vi "Configuration Dialog.vi"(8 "error in (no error)":errorcluster, 11 "Error Handler In":refnum<class "Error Handler.lvclass">) -> (0 "error out":errorcluster, 3 "Error Handler Out":refnum<class "Error Handler.lvclass">)   [LabVIEW 2020, in "Error Handler.lvclass"]
uses:
  Error Handler.lvclass
  Error Handler.lvclass/Error Handler.ctl
panel:
  in  "Silent handling?":bool
  in  "Error Log Directory":path
  in  "Cancel":bool
  in  "Commit":bool
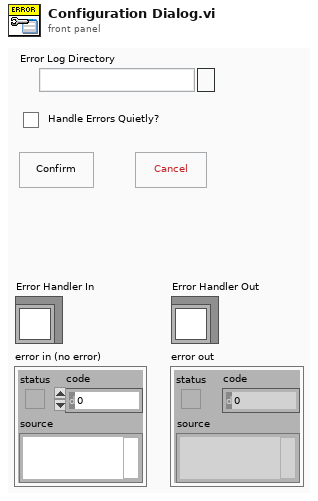
[diagram p1: front panel]
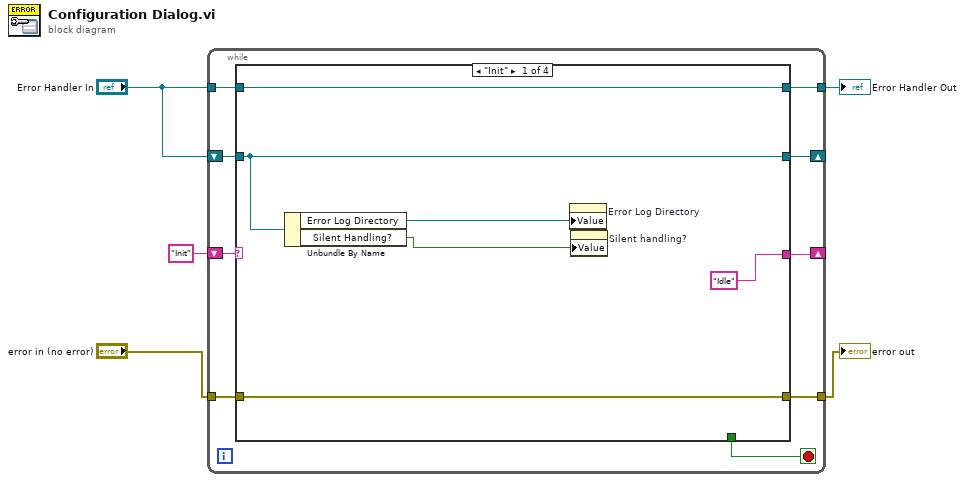
[diagram p0: block diagram]
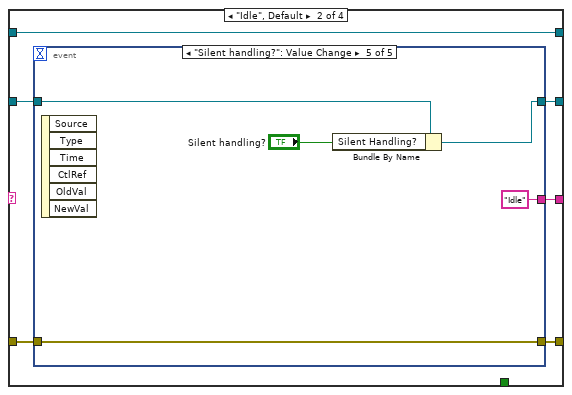
[diagram p2: hidden frame]
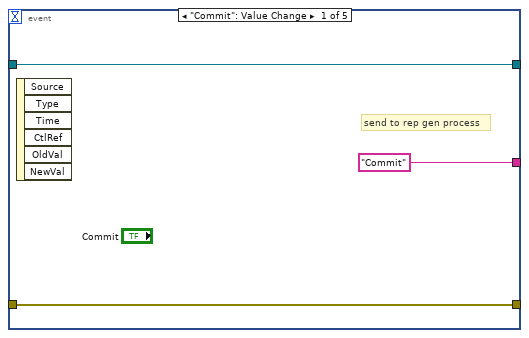
[diagram p3: hidden frame]
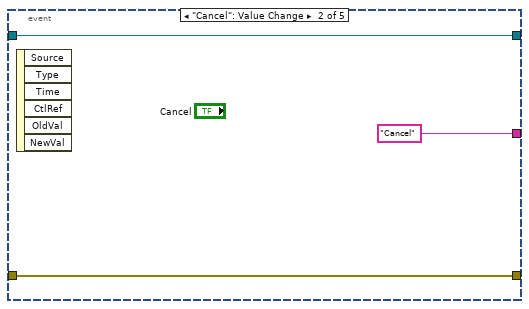
[diagram p4: hidden frame]
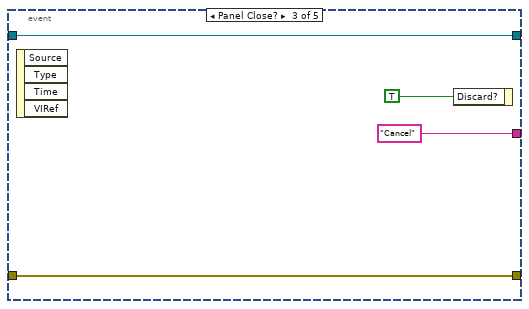
[diagram p5: hidden frame]
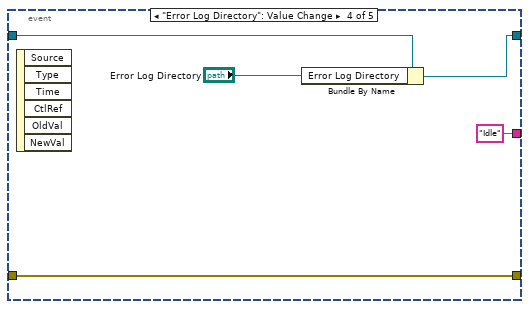
[diagram p6: hidden frame]
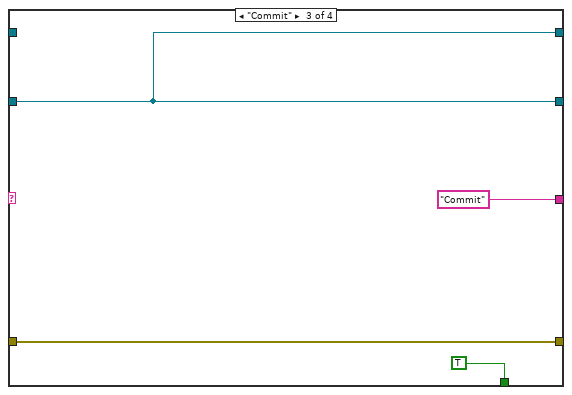
[diagram p7: hidden frame]
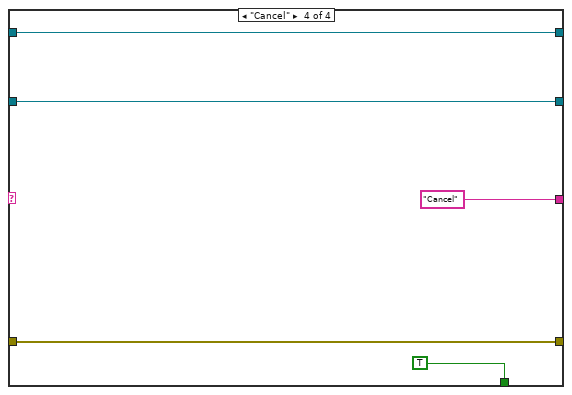
[diagram p8: hidden frame]
diagram:
  n1 = while {
    tunnel: [w14] -> w1
    tunnel: "Error Handler In" -> [w13]
    tunnel: [w12] -> w2
    tunnel: "error in (no error)" -> [w11]
    shift-right: [w8] -> _
    shift-left: "Error Handler In" -> [w9]
    shift-right: [w6] -> _
    shift-left: "Init" -> [w7]
    stop <- w10 stop-if-true
    n2 = case shown="\"Init\"" w7 {
      tunnel: [w20 w22 w50 w55] -> w14
      tunnel: w13 -> [w20 w22 _ w55]
      tunnel: [w17 w26 w49 w51] -> w12
      tunnel: w11 -> [w17 w25 w49 w51]
      tunnel: [_ _ TRUE TRUE] -> w10
      tunnel: w9 -> [w18 w24 w50 w54]
      tunnel: [w18 w23 w50 w54] -> w8
      tunnel: ["Idle" w21 "Commit" "Cancel"] -> w6
      frame "Init" {
        n3 = Unbundle By Name(w18) -> ("Error Log Directory"=w15:path, "Silent Handling?"=w16:bool)
        n4 = property on="Error Log Directory" class="Path"("Value"=w15) -> ()  [unwired: 2 in, 2 out]
        n5 = property on="Silent handling?" class="Bool (strict)"("Value"=w16) -> ()  [unwired: 2 in, 2 out]
      }
      frame "Idle", Default {
        n6 = event shown="[4] \"Silent handling?\": Value Change" {
          selector: _ -> [_ _ _ _ _]
          dyn-events: _ -> [_ _ _ _ _]
          timeout: _ -> [_ _ _ _ _]
          tunnel: [w28 w32 w36 w38 w43] -> w26
          tunnel: w25 -> [w28 w32 w36 w38 w43]
          tunnel: w24 -> [w29 w31 w35 w41 w46]
          tunnel: [w29 w31 w35 w40 w45] -> w23
          tunnel: ["Commit" "Cancel" "Cancel" "Idle" "Idle"] -> w21
          event "Commit": Value Change {
            # "send to rep gen process"
            n7 = event-data() -> ()  [unwired: 1 in, 6 out]
          }
          event "Cancel": Value Change {
            n8 = event-data() -> ()  [unwired: 1 in, 6 out]
          }
          event Panel Close? {
            n9 = event-data() -> ()  [unwired: 1 in, 4 out]
            n10 = event-data("Discard?"=TRUE) -> ()  [unwired: 1 in, 1 out]
          }
          event "Error Log Directory": Value Change {
            n11 = event-data() -> ()  [unwired: 1 in, 6 out]
            n12 = Bundle By Name(cluster=w41, "Error Log Directory"="Error Log Directory") -> (w40:refnum<class "Error Handler.lvclass">)
          }
          event "Silent handling?": Value Change {
            n13 = event-data() -> ()  [unwired: 1 in, 6 out]
            n14 = Bundle By Name(cluster=w46, "Silent Handling?"="Silent handling?") -> (w45:refnum<class "Error Handler.lvclass">)
          }
        }
      }
      frame "Commit" {
      }
      frame "Cancel" {
      }
    }
  }
  "error out" <- w2
  "Error Handler Out" <- w1
